vi "Take snapshot.vi"(9 "Right Image":T1, 11 "Left Image":T1) -> ()   [LabVIEW 2013]
uses:
  <vilib>/vision/Image Controls.llb/IMAQ Image.ctl
  Global Variables/General Globals.vi
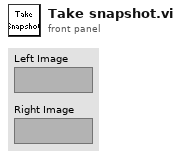
[diagram p1: front panel]
types:
  T1 = typedef "IMAQ Image.ctl" = refnum<image>
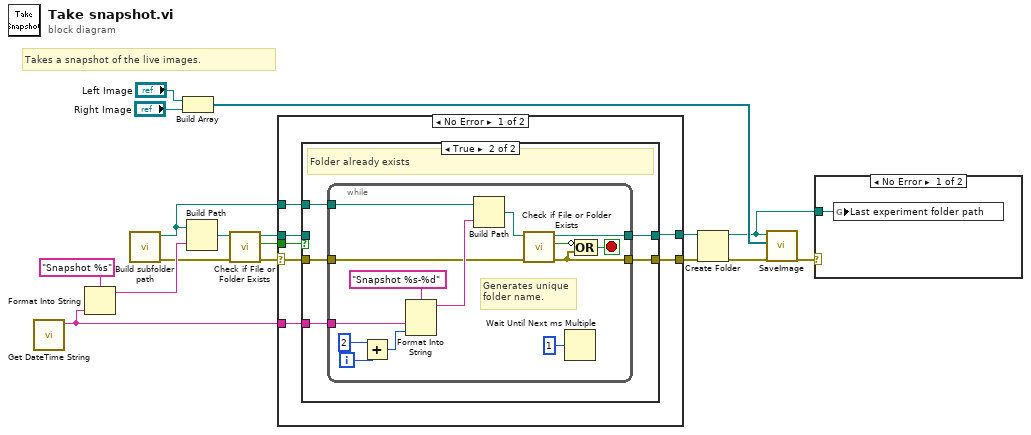
[diagram p0: block diagram]
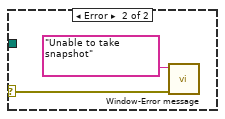
[diagram p4: hidden frame]
diagram:
  # "Takes a snapshot of the live images."
  n1 = call "Get DateTime String.vi"() -> ("date/time string"=w4:string)  [unwired: 10 in, 1 out]
  n2 = Format Into String(format string="Snapshot %s" ("name or relative path"), w4) -> (resulting string=w5:string)  [unwired: 2 in, 1 out]
  n3 = call "Build subfolder path.vi"() -> ("error out"=w1:errorcluster, "Daily folder or sub-folder path"=w2:path)  [unwired: 10 in]
  n4 = Build Array("Left Image", "Right Image") -> (w13:T1[])
  n5 = Build Path(base path=w2, name or relative path=w5) -> (appended path=w10:path)
  n6 = call <vilib>:"Check if File or Folder Exists.vi"("error in (no error)"=w1, "path"=w10) -> ("error out"=w3:errorcluster, "file or folder exists?"=w9:bool, "dup path"=w8:path)  [unwired: 7 in]
  n7 = case shown="No Error" w3 {
    selector: w3 -> [w18 w47]
    tunnel: w9 -> [w24 _]
    tunnel: w8 -> [w23 w46]
    tunnel: [w22 w46] -> w7
    tunnel: [w21 w47] -> w6
    tunnel: w2 -> [w20 _]
    tunnel: w4 -> [w19 _]
    frame No Error {
      n8 = case shown="True" w24 {
        tunnel: w23 -> [w26 _]
        tunnel: [w26 w30] -> w22
        tunnel: [w25 w28] -> w21
        tunnel: w20 -> [_ w31]
        tunnel: w19 -> [_ w29]
        tunnel: w18 -> [w25 w27]
        frame False {
          # "Folder doesn't exist"
        }
        frame True {
          # "Folder already exists"
          n9 = while {
            tunnel: w31 -> [w45]
            tunnel: [w40] -> w30
            tunnel: w29 -> [w42]
            tunnel: [w35] -> w28
            tunnel: w27 -> [w32]
            i -> [w39]
            stop <- w34 stop-if-true
            # "Generates unique\nfolder name."
            n10 = Add(x=2, y=w39) -> (x+y=w37:i32)
            n11 = Format Into String(format string="Snapshot %s-%d" ("name or relative path"), w42, w37) -> (resulting string=w43:string)  [unwired: 2 in, 1 out]
            n12 = Build Path(base path=w45, name or relative path=w43) -> (appended path=w41:path)
            n13 = call <vilib>:"Check if File or Folder Exists.vi"("error in (no error)"=w32, "path"=w41) -> ("error out"=w35:errorcluster, "file or folder exists?"=w33:bool, "dup path"=w40:path)  [unwired: 7 in]
            n14 = Wait Until Next ms Multiple(millisecond multiple=u32 1) -> ()  [unwired: 1 out]
            n15 = Compound Arithmetic op=OR(invert w33, w35) -> (w34:bool)
          }
        }
      }
    }
    frame Error {
    }
  }
  n16 = Create Folder(path (use dialog)=w7, error in=w6) -> (created path=w11:path, error out=w17:errorcluster)  [unwired: 1 in, 1 out]
  n17 = call "SaveImage.vi"("Error In"=w17, "Image In"=w13, "Snapshot images folder path"=w11) -> ("Error Out"=w12:errorcluster)  [unwired: 8 in]
  n18 = case shown="No Error" w12 {
    selector: w12 -> [_ w50]
    tunnel: w11 -> [w48 _]
    frame No Error {
      n19 = global write "General Globals.vi" "Last experiment folder path"(w48) -> ()
    }
    frame Error {
      n20 = call "Window-Error message.vi"("error in (no error)"=w50, "Message"="Unable to take snapshot") -> ()  [unwired: 9 in, 1 out]
    }
  }
